vi "defer panel updates step2.vi"(8 "error in (no error)":errorcluster, 11 "Refs":T1) -> (0 "error out":errorcluster)   [LabVIEW 2020, in "Defer Panel Updates OpenSource.lvlib"]
doc: "This VI will turn off front panel deferment if and only if the step1 turned this on.\n\nThe intent is for this toolkit to be used in a nested manner"
uses:
  Defer Panel Updates OpenSource.lvlib
  defer panel updates data.ctl
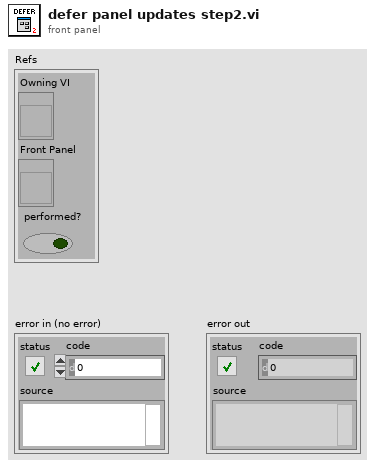
[diagram p1: front panel]
types:
  T1 = typedef "Defer Panel Updates OpenSource.lvlib/defer panel updates data.ctl" = cluster{"Owning VI":refnum<vi>, "Front Panel":refnum<vi>, "performed?":bool}
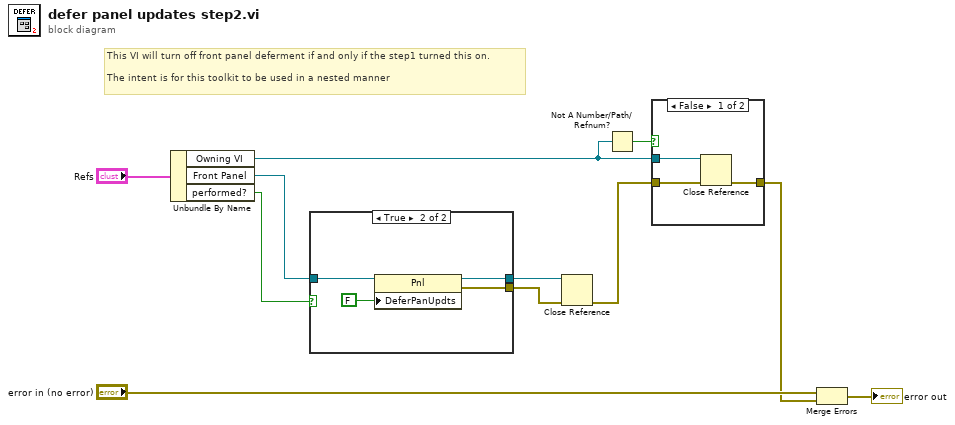
[diagram p0: block diagram]
diagram:
  # "This VI will turn off front panel deferment if and only if the step1 turned this on.\n\nThe intent is for this toolkit to be used in a nested manner"
  n1 = Unbundle By Name("Refs") -> ("Owning VI"=w6:refnum<vi>, "Front Panel"=w7:refnum<vi>, "performed?"=w1:bool)
  n2 = case shown="True" w1 {
    tunnel: [w12 w15] -> w10
    tunnel: [_ w14] -> w9
    tunnel: w7 -> [w12 w13]
    frame False {
    }
    frame True {
      n3 = property class="Pnl"(reference=w13, "DeferPanUpdts"=FALSE ("Defer Panel Updates")) -> (reference out=w15:refnum<vi>, error out=w14:errorcluster)  [unwired: 1 in]
    }
  }
  n4 = Close Reference(reference=w10, error in (no error)=w9) -> (error out=w11:errorcluster)
  n5 = Not A Number/Path/Refnum?(number/path/refnum=w6) -> (NaN/Path/Refnum?=w5:bool)
  n6 = case shown="False" w5 {
    tunnel: w11 -> [w19 w20]
    tunnel: w6 -> [w18 _]
    tunnel: [w17 w20] -> w3
    frame False {
      n7 = Close Reference(reference=w18, error in (no error)=w19) -> (error out=w17:errorcluster)
    }
    frame True {
    }
  }
  n8 = Merge Errors("error in (no error)", w3) -> (→"error out":errorcluster)
